vi "Trim Prefix.vi"(10 "Prefix":string, 11 "String":string) -> (3 "String":string)   [LabVIEW 2011, in "LVH-Toolbox.lvlib" / "LVH-SystemTools.lvlib"]
doc: "Check if string contains specified prefix. If so remove it and return remaining string."
uses:
  LVH-SystemTools.lvlib
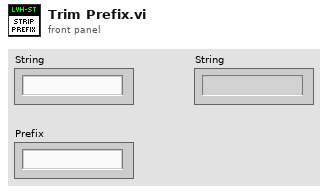
[diagram p1: front panel]
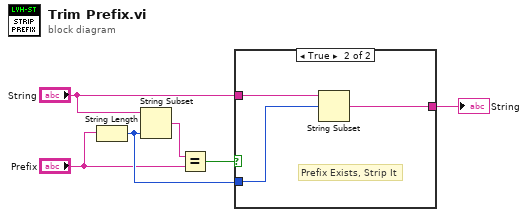
[diagram p0: block diagram]
diagram:
  n1 = String Length(string="Prefix") -> (length=w4:i32)
  n2 = String Subset(string="String", length (rest)=w4) -> (substring=w6:string)  [unwired: 1 in]
  n3 = Equal?(x=w6, y="Prefix") -> (x = y?=w5:bool)
  n4 = case shown="True" w5 {
    tunnel: "String" -> [w7 w10]
    tunnel: w4 -> [_ w9]
    tunnel: [w7 w8] -> w2
    frame False {
      # "Prefix DNE,\n Nothing To Do Here...."
    }
    frame True {
      # "Prefix Exists, Strip It"
      n5 = String Subset(string=w10, offset (0)=w9) -> (substring=w8:string)  [unwired: 1 in]
    }
  }
  "String" <- w2
